vi "Flush Buffer.vi"(8 "error in":errorcluster, 10 "return elements(T)":bool=TRUE, 11 "Buffer in":refnum<data-value>) -> (0 "error out":errorcluster, 2 "elements":variant[](array[variant]), 3 "Buffer":refnum<data-value>)   [LabVIEW 2013, in "CircularBuffer.lvlib" / "VariantBuffer.lvclass"]
doc: "This VI returns data from the ring buffer starting from the oldest data and ending with the newest.\n\nThe data is duplicated at the output so this VI allocates new place in the memory for the output."
uses:
  VariantBuffer.lvclass
  VariantBuffer.lvclass/VariantBuffer.ctl
  buffer-event -- enum.ctl
  WriteBufferError.vi
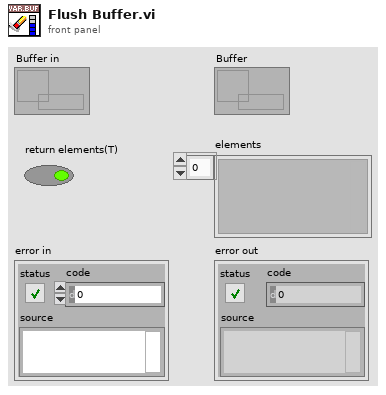
[diagram p1: front panel]
types:
  T1 = typedef "CircularBuffer.lvlib/VariantBuffer.lvclass/buffer-event -- enum.ctl" = enum16{"element-added", "element-removed", "filled", "emptied", "resized", "default-changed", "destroyed"}
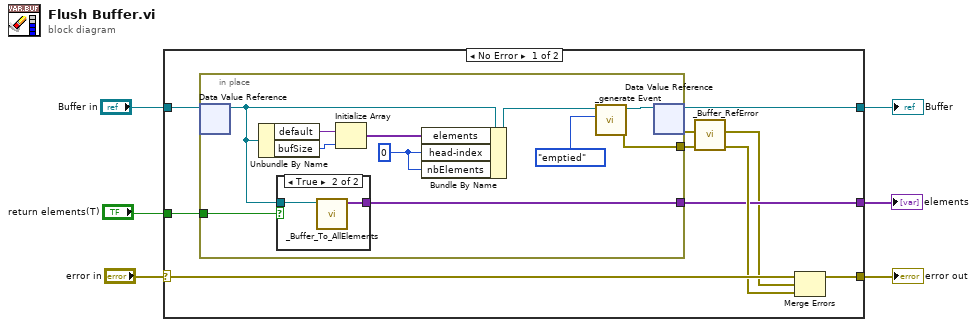
[diagram p0: block diagram]
diagram:
  n1 = case shown="No Error" "error in" {
    selector: "error in" -> [w13 w29]
    tunnel: "Buffer in" -> [w14 w30]
    tunnel: [w12 w30] -> w5
    tunnel: [w15 w29] -> w2
    tunnel: [w10 _] -> w4
    tunnel: "return elements(T)" -> [w9 _]
    frame No Error {
      n2 = in-place {
        in-place-border: [w19] -> w11
        in-place-border: [w17] -> w10
        in-place-border: w9 -> [w16]
        w25 = 0 ("Index")
        n3 = in-place-dvr #1(w14) -> (w18:refnum<class "VariantBuffer.lvclass">)  [unwired: 1 out]
        n4 = Unbundle By Name(w18) -> ("default"=w23:variant, "bufSize"=w24:i32)
        n5 = case shown="True" w16 {
          tunnel: w18 -> [_ w28]
          tunnel: [_ w27] -> w17
          frame False {
          }
          frame True {
            n6 = call "_Buffer_To_AllElements.vi"("Buffer"=w28) -> ("elements"=w27:variant[])  [unwired: 10 in]
          }
        }
        n7 = Initialize Array(w23, w24) -> (w26:variant[])
        n8 = Bundle By Name(cluster=w18, "elements"=w26, "head-index"=w25, "nbElements"=w25) -> (w21:refnum<class "VariantBuffer.lvclass">)
        n9 = call "_generate Event.vi"("event"=buffer-event_--_enum."emptied", "VariantBuffer"=w21) -> ("error out"=w19:errorcluster, "VariantBuffer out"=w20:refnum<class "VariantBuffer.lvclass">)  [unwired: 8 in]
        n10 = in-place-dvr #1(w20) -> (w12:refnum<data-value>, w8:errorcluster)
      }
      n11 = call "_Buffer_RefError.vi"("error in (no error)"=w8) -> ("error out"=w7:errorcluster)  [unwired: 10 in]
      n12 = Merge Errors(w13, w7, w11) -> (w15:errorcluster)
    }
    frame Error {
    }
  }
  "error out" <- w2
  "Buffer" <- w5
  "elements" <- w4
